vi "cycle writer.vi"(7 "wheel name":path=path "C:/Documents and Settings/Administrator/Desktop/data acquisition 2009/sub vis/wheel creation/cycle results default.txt", 8 "error in":errorcluster, 10 "Cycle data":string="0.000000\t0.000000\t0.000000\t0.000000\t0.000000\t0.993919\t0.166802\t1.000000\t0.068912\t0.000000\tInf\tNaN\t0.000000\t0.000000\t0.000000\t0.000000\r\n", 11 "Wheel data":string="3\t45558\tcaffee\tstandard\ts\t5000\t1\tfinished\r\n") -> (0 "error out":errorcluster={"status"=TRUE, "code"=1430, "source"="Open/Create/Replace File in cycle writer.vi->2d ams run.vi<APPEND>\n"}, 3 "readouts string":string)   [LabVIEW 2016]
doc: "This vi allows the boiler program to keep a log file that can be viewed later. It checks to see if the boiler log.txt exsits, and creates one in the same folder as this vi."
uses:
  realtime data/pixie vis/controls/header name control.ctl
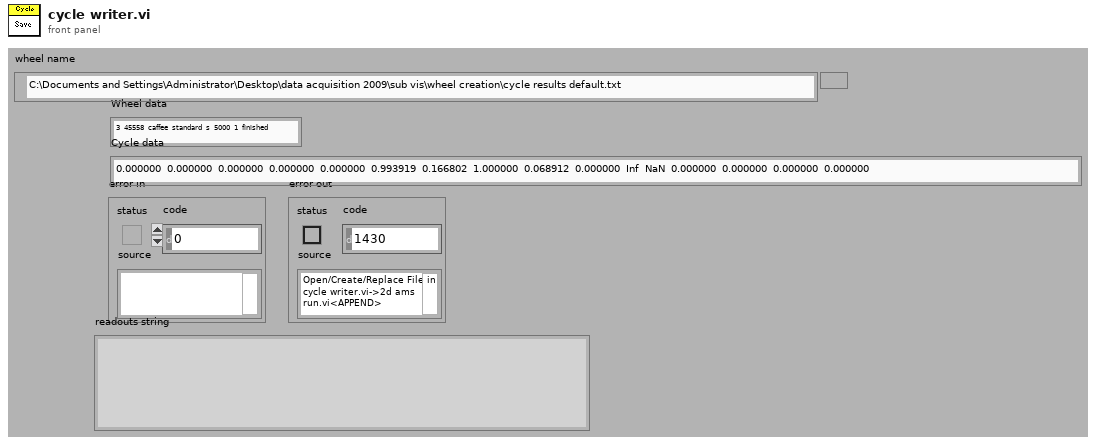
[diagram p1: front panel]
types:
  T1 = typedef "header name control.ctl" = string
  T2 = enum16{"open", "replace", "create", "open or create", "replace or create", "replace or create with confirmation"}
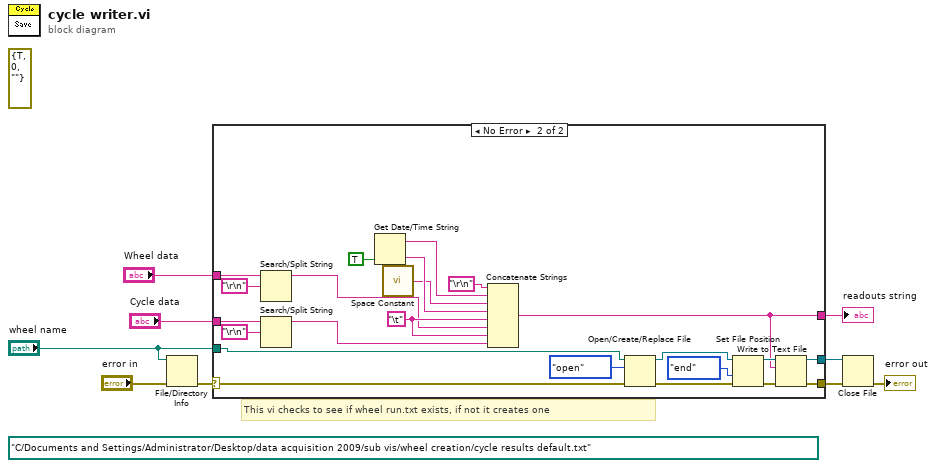
[diagram p0: block diagram]
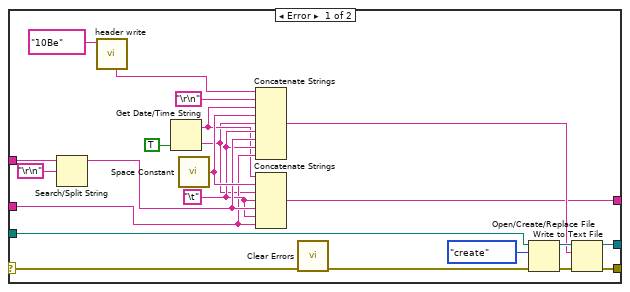
[diagram p2: hidden frame]
diagram:
  (unwired) errorcluster {"status"=TRUE, "code"=0, "source"=""} ("error IO")
  (unwired) path "C:/Documents and Settings/Administrator/Desktop/data acquisition 2009/sub vis/wheel creation/cycle results default.txt" ("path")
  # "This vi checks to see if wheel run.txt exists, if not it creates one"
  n1 = File/Directory Info(path="wheel name", error in="error in") -> (error out=w1:errorcluster)  [unwired: 6 out]
  n2 = case shown="No Error" w1 {
    selector: w1 -> [w25 w52]
    tunnel: "wheel name" -> [w28 w51]
    tunnel: "Wheel data" -> [w22 w39]
    tunnel: "Cycle data" -> [w14 w35]
    tunnel: [w27 w45] -> w6
    tunnel: [w26 w40] -> w5
    tunnel: [w13 w32] -> w2
    frame Error {
      w15 = "\t" ("string")
      n3 = Search/Split String(string=w22, search string/char (-)="\r\n") -> (substring before match=w16:string)  [unwired: 1 in, 2 out]
      n4 = call "header write.vi"("Which header name"=T1 "10Be") -> ("name output"=w21:string)  [unwired: 10 in]
      n5 = Get Date/Time String(want seconds? (F)=TRUE) -> (date string=w11:string, time string=w10:string)  [unwired: 2 out]
      n6 = call <vilib>:"Space Constant.vi"() -> ("String"=w17:string)
      n7 = Concatenate Strings(w21, "\r\n", w11, w17, w10, w15, w16, w15, w14) -> (w20:string)
      n8 = Concatenate Strings(w11, w17, w10, w15, w16, w15, w14) -> (w13:string)
      n9 = call <vilib>:"Clear Errors.vi"("error in (no error)"=w25) -> ("error out"=w24:errorcluster)  [unwired: 1 in, 5 out]
      n10 = Open/Create/Replace File(file path (use dialog)=w28, error in=w24, operation (0:open)=T2."create") -> (refnum out=w30:refnum<file>, error out=w31:errorcluster)  [unwired: 1 in, 3 out]
      n11 = Write to Text File(file (use dialog)=w30, text=w20, error in=w31) -> (refnum out=w26:refnum<file>, error out=w27:errorcluster)  [unwired: 2 out]
    }
    frame No Error {
      w53 = "\t" ("string")
      n12 = Search/Split String(string=w39, search string/char (-)="\r\n") -> (substring before match=w37:string)  [unwired: 1 in, 2 out]
      n13 = Search/Split String(string=w35, search string/char (-)="\r\n") -> (substring before match=w34:string)  [unwired: 1 in, 2 out]
      n14 = Get Date/Time String(want seconds? (F)=TRUE) -> (date string=w43:string, time string=w42:string)  [unwired: 2 out]
      n15 = call <vilib>:"Space Constant.vi"() -> ("String"=w41:string)
      n16 = Concatenate Strings("\r\n", w43, w41, w42, w53, w37, w53, w34) -> (w32:string)
      n17 = Open/Create/Replace File(file path (use dialog)=w51, error in=w52, operation (0:open)=T2."open") -> (refnum out=w49:refnum<file>, error out=w50:errorcluster)  [unwired: 4 out]
      n18 = Set File Position(refnum=w49, from (0:start)=enum16{"start", "end", "current"}."end", error in=w50) -> (refnum out=w46:refnum<file>, error out=w47:errorcluster)  [unwired: 1 out]
      n19 = Write to Text File(file (use dialog)=w46, text=w32, error in=w47) -> (refnum out=w40:refnum<file>, error out=w45:errorcluster)  [unwired: 2 out]
    }
  }
  "readouts string" <- w2
  n20 = Close File(refnum=w5, error in=w6) -> (error out=→"error out":errorcluster)  [unwired: 1 out]
